vi "QuadratureCtr_X4.vi"(7 "Direction?":bool=TRUE, 8 "First Run?":bool, 9 "Reset":bool, 10 "Source B":bool, 11 "Source A":bool) -> (2 "Position":i32)   [LabVIEW 2014, in "SYSID.lvlib"]
doc: "This VI implements a quadrature counter. It computes position using digital signals A and B of a quadrature encoder. It was designed to be called as a subVI in a loop on a LabVIEW FPGA VI block diagram.\n\nThis VI is marked as reentrant so that it can be placed multiple times on the block diagram. Duplicate logic will be created in the FPGA for each instance of this VI the block diagram.\n\n<B>Inputs:</B>\n<B>Source A</B> - This is digital signal A from a quadrature encoder.\n\n<B>Source B</B> - This is digital signal B from a quadrature encoder.\n\n<B>Direction?</B> - This control determines whether the position increments or decrements as edges are dectected on A and B. If Direction? is TRUE, then the position increments when signal A leads B and decrements when signal B leads A. If Direction? is FALSE, then the position increments when signal B leads A and decrements when signal A leads B.\n\n<B>Reset</B> - This control resets the quadrature counter. When a TRUE is written to Reset, the position value is reset to zero.\n\n<B>First Run?</B> - This control ensures that the quadrature counter's initial position is zero. The caller of this VI should wire a TRUE into this input for its first call and a FALSE for subsequent calls.\n\n<B>Outputs:</B>\n<B>Position</B> - This is the position of the quadrature counter. It represents the position of the counter since it was started or since it was last reset."
uses:
  SYSID.lvlib
  <vilib>/rvi/Emulation/niFpgaSctlEmulationGetInTimedLoop.vi
  <vilib>/rvi/Emulation/niFpgaProcessEmulError.vi
panel:
  out "B register":bool
  out "A register":bool
  # "Inputs"
  # "Registers"
  # "Outputs"
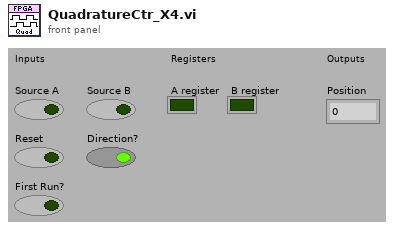
[diagram p1: front panel]
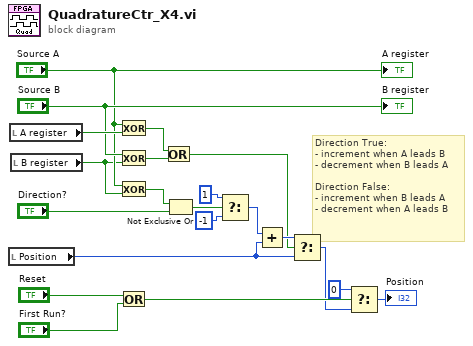
[diagram p0: block diagram]
diagram:
  # "Direction True:\n- increment when A leads B\n- decrement when B leads A\n\nDirection False:\n- increment when B leads A\n- decrement when A leads B"
  n1 = local read "Position"() -> (w6:i32)
  n2 = local read "A register"() -> (w16:bool)
  n3 = local read "B register"() -> (w11:bool)
  n4 = Exclusive Or(1:w16, 2:"Source A") -> (0:w14:bool)
  n5 = Exclusive Or(1:w11, 2:"Source B") -> (0:w13:bool)
  n6 = Exclusive Or(1:w11, 2:"Source A") -> (0:w3:bool)
  n7 = Or(x="Reset", y="First Run?") -> (x .or. y?=w19:bool)
  n8 = Or(x=w14, y=w13) -> (x .or. y?=w4:bool)
  n9 = Not Exclusive Or(1:"Direction?", 2:w3) -> (0:w1:bool)
  n10 = Select(t=1 ("I32"), s=w1, f=-1 ("I32")) -> (s? t:f=w5:i32)
  n11 = Add(x=w5, y=w6) -> (x+y=w7:i32)
  n12 = Select(t=w7, s=w4, f=w6) -> (s? t:f=w17:i32)
  n13 = Select(t=0 ("I32"), s=w19, f=w17) -> (s? t:f=→"Position":i32)
  "A register" <- "Source A"
  "B register" <- "Source B"
